vi "UIMessage Callback Error Handler.vi"(8 "error in (no error)":errorcluster, 9 "TSnax:UIMessage":refnum<class "UIMessage.lvclass">, 10 "VI":T1, 11 "TSnax:Engine":refnum<class "Engine.lvclass">) -> ()   [LabVIEW 2020, in "TSnax.lvlib" / "Engine.lvclass"]
uses:
  Engine.lvclass
  UIMessage/UIMessage.lvclass
  Engine.lvclass/Engine.ctl
  UIMsg Callback VI.ctl
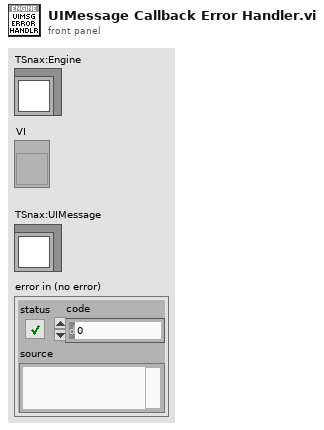
[diagram p1: front panel]
types:
  T1 = typedef "TSnax.lvlib/Engine.lvclass/UIMsg Callback VI.ctl" = refnum<vi>
  T2 = typedef "TSnax.lvlib/UIMsg.ctl" = enum16{"Unknown", "BreakOnUserRequest", "BreakOnBreakpoint", "BreakOnRunTimeError", "Trace", "TerminatingExecution", "AbortingExecution", "KillingExecutionThreads", "EndExecution", "ShutDownComplete", "StartExecution", "ProgressPercent", "ProgressText", "StartInteractiveExecution", "EndInteractiveExecution", "TerminatingInteractiveExecution", "TerminationCancelled", "ResumeFromBreak", "StartFileExecution", "EndFileExecution", "ShutDownCancelled", "LocalizationSettingChanged", "OpenWindows", "TileWindows", "CascadeWindows", "ReportChanged", "CloseWindows", "RefreshWindows", "ClientFileChanged", "DisplayReport", "ModelState_Initializing", "ModelState_Waiting", "ModelState_Identified", "ModelState_BeginTesting", "ModelState_TestingComplete", "ModelState_PostProcessingComplete", "ModelState_EnabledStateSet", "ReportLocationChanged", "GotoLocation", "PushUndoItem", "OutputMessages", "TypePaletteFileListChanged", "NonTerminatingThreadsArePreventingTermination", "ModelState_PostProcessing", "ReportCollectionChanged", "RuntimeError"}
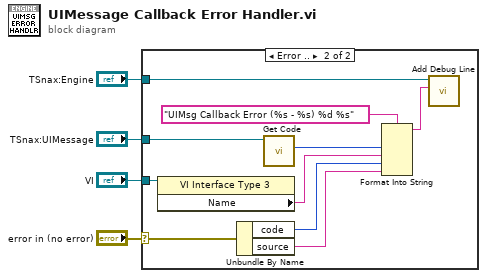
[diagram p0: block diagram]
diagram:
  n1 = case shown="Error .." "error in (no error)" {
    selector: "error in (no error)" -> [_ w9]
    tunnel: "VI" -> [_ w14]
    tunnel: "TSnax:UIMessage" -> [_ w13]
    tunnel: "TSnax:Engine" -> [_ w6]
    frame No Error {
    }
    frame Error {
      n2 = property class="VI Interface Type 3"(reference=w14) -> ("Name"=w10:string)  [unwired: 1 in, 2 out]
      n3 = Unbundle By Name(w9) -> ("code"=w8:i32, "source"=w7:string)
      n4 = call "Get Code.vi"("UIMessage in"=w13) -> ("Code"=w12:T2)  [unwired: 8 in, 2 out]
      n5 = Format Into String(format string="UIMsg Callback Error (%s - %s) %d %s", w12, w10, w8, w7) -> (resulting string=w5:string)  [unwired: 2 in, 1 out]
      n6 = call "Add Debug Line.vi"("Debug Line"=w5, "Engine in"=w6) -> ()  [unwired: 10 in]
    }
  }
